vi "Write socket.vi"(6 "ms timeout listening":i32, 8 "error in (no error)":errorcluster, 9 "port":u16, 10 "ip":string="localhost", 11 "Server in":refnum<class "TCP-Server.lvclass">) -> (0 "error out":errorcluster, 3 "Server out":refnum<class "TCP-Server.lvclass">)   [LabVIEW 2018, in "TCP-Server.lvclass"]
uses:
  TCP-Server.lvclass
  TCP-Server.lvclass/TCP-Server.ctl
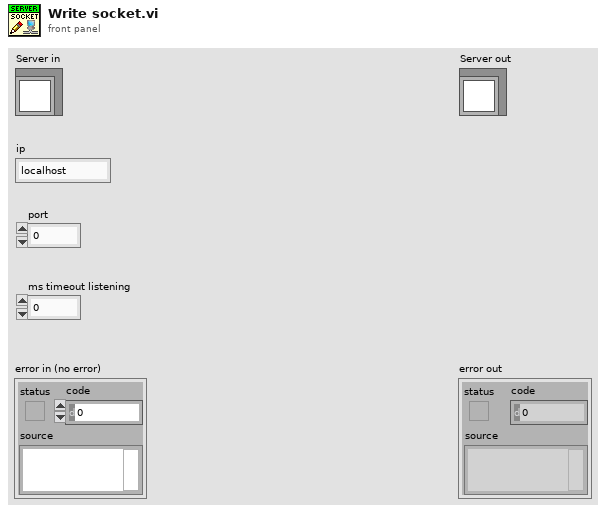
[diagram p1: front panel]
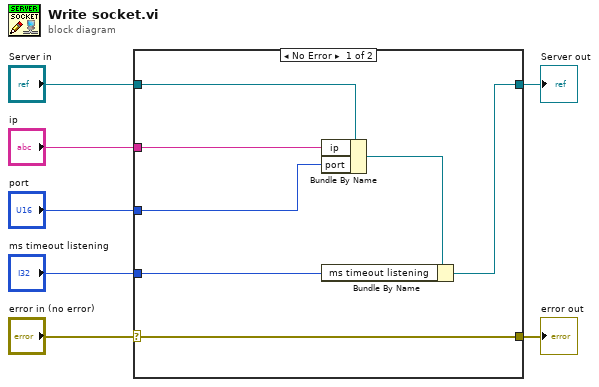
[diagram p0: block diagram]
diagram:
  n1 = case shown="No Error" "error in (no error)" {
    selector: "error in (no error)" -> [w14 w15]
    tunnel: [w14 w15] -> w6
    tunnel: [w9 w16] -> w4
    tunnel: "Server in" -> [w13 w16]
    tunnel: "ip" -> [w12 _]
    tunnel: "port" -> [w11 _]
    tunnel: "ms timeout listening" -> [w8 _]
    frame No Error {
      n2 = Bundle By Name(cluster=w13, "ip"=w12, "port"=w11) -> (w10:refnum<class "TCP-Server.lvclass">)
      n3 = Bundle By Name(cluster=w10, "ms timeout listening"=w8) -> (w9:refnum<class "TCP-Server.lvclass">)
    }
    frame Error {
    }
  }
  "error out" <- w6
  "Server out" <- w4
